vi "2023_day18.vi"() -> ()   [LabVIEW 2021]
panel:
  out "Task 2":i64
  out "Task 1 Data":cluster{i64[], i64[]}(graph)
  out "Task 2 Data":cluster{i64[], i64[]}(graph)
  out "Task 1":i64
  in  "Switch":bool caption="Ex. Data  vs.  User Data"
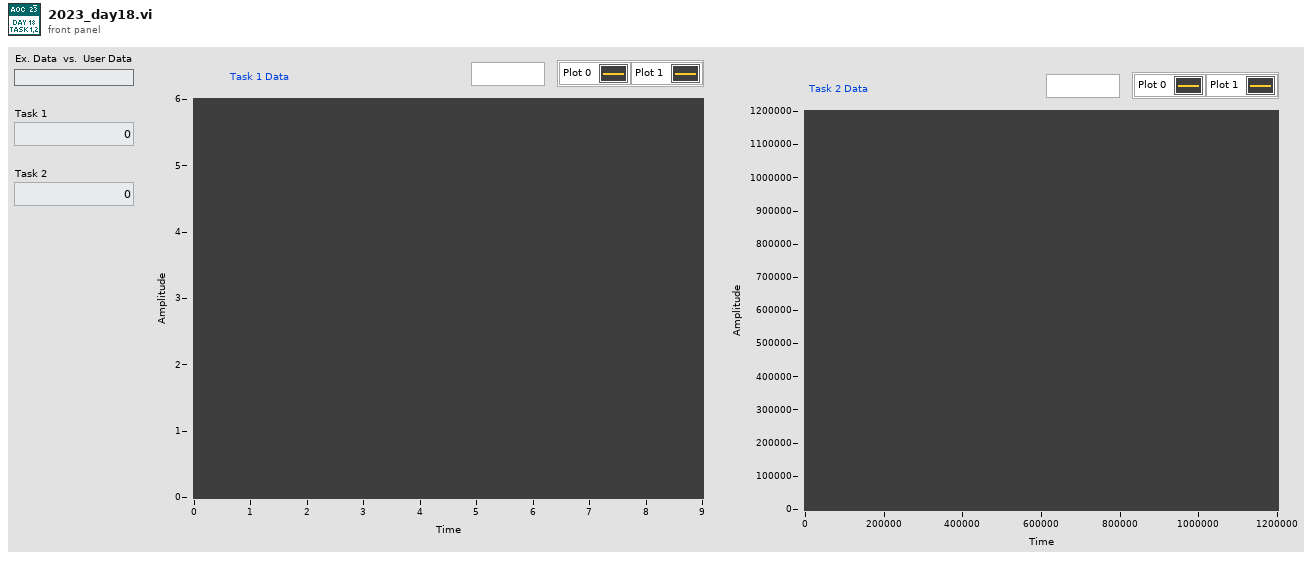
[diagram p1: front panel]
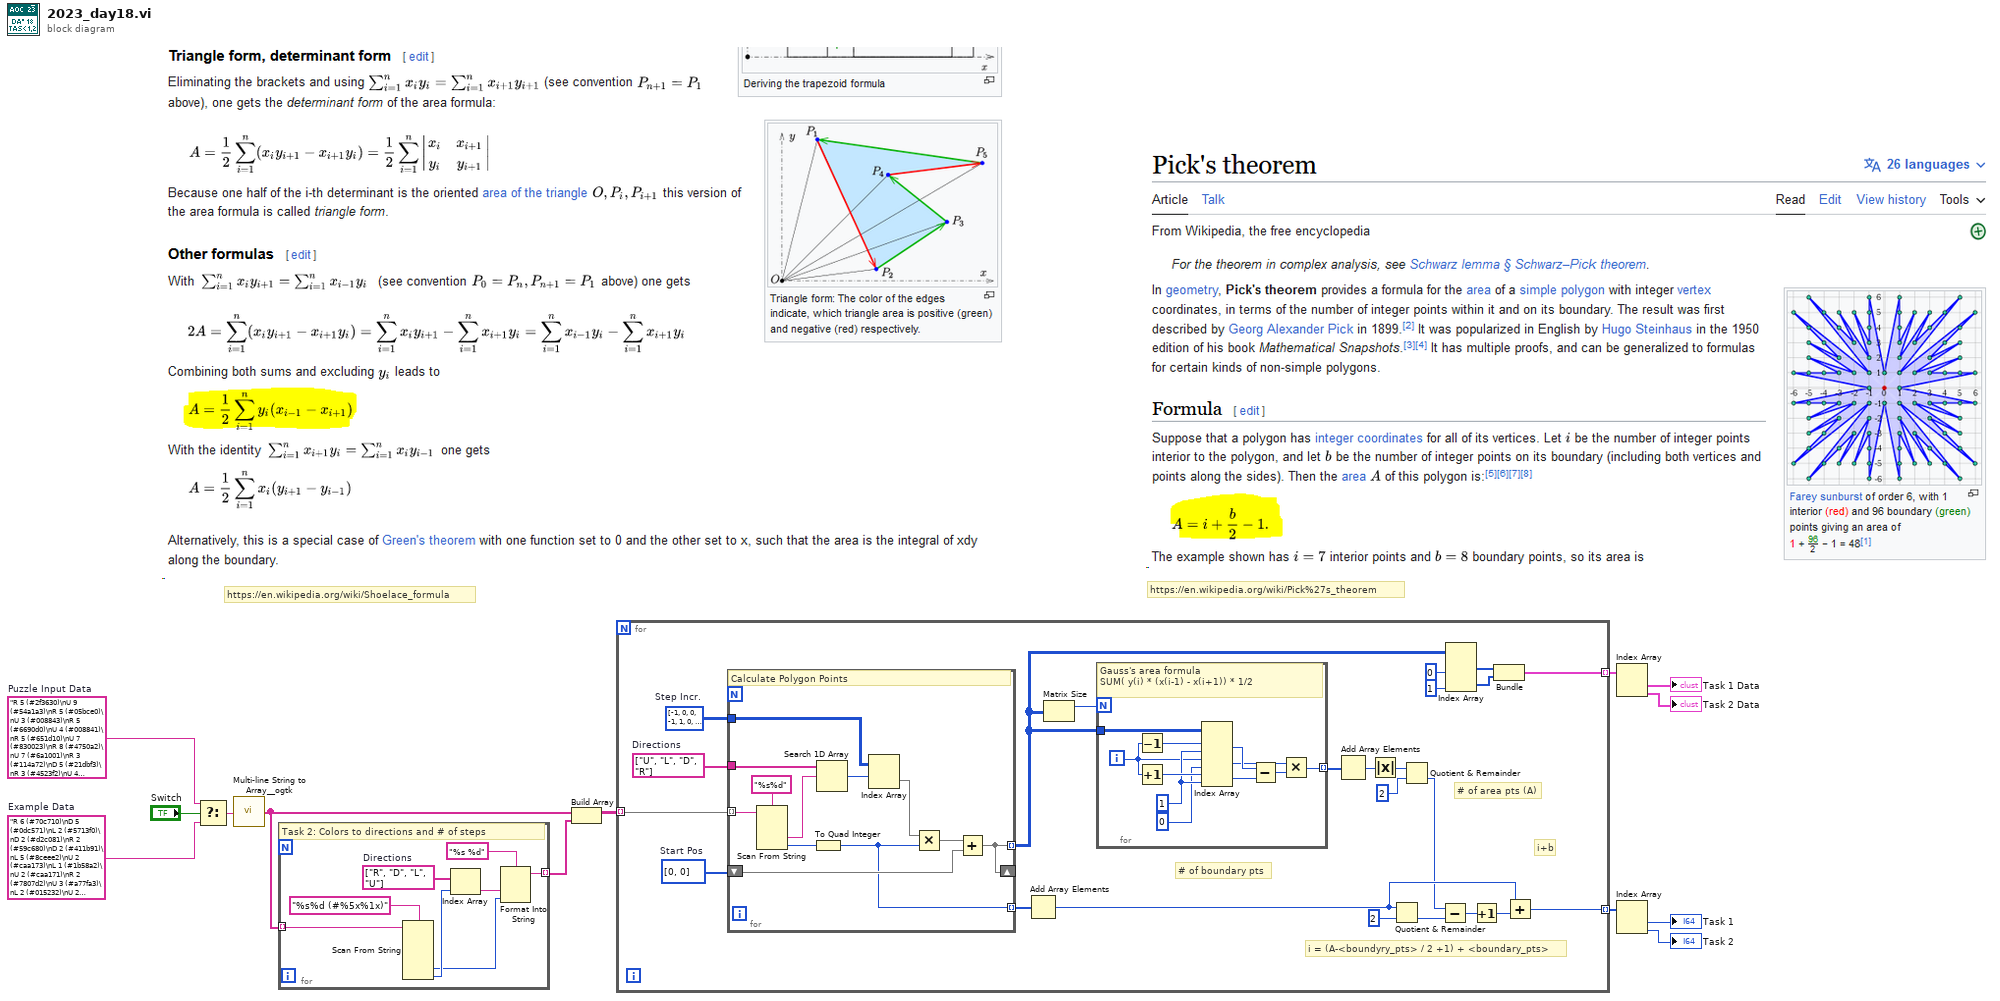
[diagram p0: block diagram]
diagram:
  w12 = "R 5 (#2f3630)\nU 9 (#54a1a3)\nR 5 (#05bce0)\nU 3 (#008843)\nR 5 (#6690d0)\nU 4 (#008841)\nR 5 (#651d10)\nU 7 (#830023)\nR 8 (#4750a2)\nU 7 (#6a1001)\nR 3 (#114a72)\nD 5 (#21dbf3)\nR 3 (#4523f2)\nU 4 (#3a1e43)\nR 4 (#2eef10)\nD 4 (#352183)\nR 5 (#2eef12)\nD 6 (#1fd943)\nL 7 (#5c0bd2)\nD 5 (#32d3b1)\nL 5 (#47d3d0)\nD 3 (#3032e1)\nR 2 (#47d3d2)\nD 4 (#4dee61)\nR 4 (#044a92)\nD 4 (#494b23)\nR 2 (#132772)\nD 3 (#2186a3)\nR 7 (#49e542)\nU 3 (#864783)\nR 3 (#3afdd2)\nU 5 (#2ab8d1)\nR 6 (#2d5072)\nD 5 (#362ab1)\nR 4 (#2d5070)\nU 5 (#46eaa1)\nR 9 (#183c12)\nU 3 (#494b21)\nR 3 (#584d32)\nU 4 (#6a1003)\nR 3 (#618682)\nU 4 (#5a1853)\nR 6 (#30cf00)\nU 6 (#6b3a23)\nR 5 (#5e1260)\nU 2 (#20b7d3)\nR 3 (#1d2ec0)\nU 10 (#89f613)\nR 5 (#16c5b0)\nU 3 (#26b1d3)\nR 4 (#475e70)\nU 3 (#007223)\nR 5 (#3cf870)\nU 3 (#851f83)\nR 8 (#326e40)\nU 5 (#043ad3)\nR 4 (#2eb0a0)\nU 5 (#26e791)\nR 3 (#0b6950)\nU 7 (#323af1)\nL 3 (#0b6952)\nU 3 (#4ffc41)\nL 4 (#721f70)\nU 8 (#0137b1)\nR 4 (#5c9d22)\nU 3 (#55ff21)\nR 5 (#5c9d20)\nU 3 (#3b2d71)\nR 5 (#721f72)\nU 7 (#1fa921)\nR 8 (#3012f0)\nD 5 (#4c6a91)\nR 8 (#61af70)\nD 4 (#4c6a93)\nR 6 (#2e21b0)\nD 2 (#7df243)\nR 2 (#108f72)\nD 9 (#239da3)\nR 5 (#1f8fb0)\nD 8 (#8e8b71)\nR 5 (#5a6f50)\nD 2 (#8e8b73)\nR 3 (#159190)\nD 5 (#5f70a3)\nL 5 (#012372)\nD 3 (#04bf23)\nL 5 (#72bbe2)\nD 6 (#04bf21)\nL 3 (#1bb142)\nD 3 (#0f6693)\nL 4 (#108f70)\nD 6 (#0ecae3)\nL 6 (#407170)\nD 8 (#10ff11)\nL 7 (#18f910)\nD 6 (#10ff13)\nR 2 (#483d30)\nD 6 (#30a891)\nR 4 (#1ed8b0)\nD 5 (#688901)\nR 4 (#130de0)\nD 6 (#4d20e1)\nR 5 (#4b1000)\nU 7 (#877bf1)\nR 2 (#395410)\nU 4 (#877bf3)\nR 4 (#167f10)\nD 2 (#486f11)\nR 7 (#54e8d0)\nD 2 (#504301)\nR 2 (#8035e2)\nD 7 (#433471)\nR 3 (#8035e0)\nD 3 (#26cad1)\nR 3 (#4b3dc0)\nD 5 (#802d11)\nR 2 (#05af00)\nD 4 (#3b3f31)\nR 5 (#0dfed0)\nD 8 (#3b4341)\nL 6 (#489830)\nD 3 (#3b4343)\nL 3 (#4e0bd0)\nD 7 (#0f7fd1)\nR 6 (#1c6dd0)\nD 2 (#318d21)\nR 3 (#0cb8f2)\nD 6 (#68acd1)\nR 2 (#432822)\nD 3 (#218ee1)\nR 11 (#661ec2)\nU 3 (#218ee3)\nR 5 (#0b10d2)\nU 4 (#2233f1)\nL 3 (#2a5330)\nU 3 (#0df7d1)\nL 9 (#5ff680)\nU 4 (#2b9701)\nR 12 (#8b68d0)\nU 3 (#2b9703)\nL 5 (#086f10)\nU 7 (#1f1431)\nR 4 (#6937b0)\nU 5 (#2cce51)\nR 3 (#26cb50)\nD 8 (#3ee1c1)\nR 6 (#3c8a40)\nD 5 (#7e7211)\nR 7 (#7190e0)\nD 3 (#036101)\nR 6 (#6110b0)\nD 3 (#89da01)\nL 12 (#1f2cc0)\nD 3 (#2b7181)\nL 4 (#3942b0)\nD 5 (#10f821)\nL 2 (#61ae90)\nD 6 (#04dee1)\nL 6 (#2fc950)\nD 2 (#04dee3)\nL 8 (#353d90)\nD 4 (#1e21b1)\nL 3 (#46fa00)\nD 4 (#3ea393)\nR 5 (#5c2e32)\nD 5 (#361be3)\nR 6 (#2ddc12)\nU 4 (#4b1a83)\nR 6 (#135722)\nU 6 (#521483)\nR 9 (#7382b2)\nD 6 (#239da3)\nR 3 (#3ed420)\nD 4 (#3a0c73)\nR 6 (#5a68d0)\nD 3 (#76f053)\nL 5 (#244ec0)\nD 4 (#062573)\nL 8 (#053c50)\nD 5 (#0bfac3)\nR 3 (#123e30)\nD 7 (#21c2c3)\nR 6 (#0b11b0)\nD 3 (#6781f3)\nR 9 (#720e70)\nD 3 (#7ddd13)\nL 11 (#33d6f0)\nD 2 (#1b2d83)\nL 7 (#5f0280)\nD 5 (#579183)\nR 4 (#5f0282)\nD 6 (#5c9303)\nR 3 (#3c6770)\nD 4 (#2b6333)\nR 5 (#4f28a0)\nU 5 (#55d573)\nR 6 (#2b03a0)\nU 5 (#244bd3)\nR 5 (#644122)\nU 7 (#08ab63)\nR 7 (#232bc2)\nU 5 (#71f5e3)\nR 4 (#060d22)\nU 3 (#168c63)\nR 4 (#44efa2)\nD 3 (#17c163)\nR 9 (#2ed822)\nD 6 (#17c161)\nR 10 (#4b9682)\nD 6 (#168c61)\nR 6 (#1ab282)\nD 3 (#490b43)\nL 6 (#639022)\nD 4 (#447151)\nL 5 (#0596c0)\nU 4 (#2fba61)\nL 5 (#0596c2)\nD 4 (#201131)\nL 3 (#1f9c52)\nD 3 (#0c4a23)\nR 9 (#266412)\nD 3 (#68bea3)\nR 7 (#266410)\nD 4 (#1f3423)\nR 3 (#51d9c2)\nD 6 (#1f6633)\nR 8 (#7382b0)\nU 8 (#01fca3)\nR 7 (#3271f0)\nU 4 (#7ee903)\nR 6 (#581210)\nD 7 (#7ee901)\nR 2 (#12dd60)\nU 7 (#15a1a3)\nR 6 (#7c30f0)\nU 2 (#591961)\nR 3 (#69efd0)\nU 4 (#591963)\nL 9 (#32e7e0)\nU 3 (#574071)\nL 3 (#50c6a0)\nU 3 (#0be261)\nL 5 (#6ae5c0)\nU 3 (#5c08b1)\nL 3 (#7158d0)\nU 2 (#36fe01)\nL 4 (#325c22)\nU 9 (#305be1)\nR 3 (#325c20)\nU 2 (#36c0a1)\nR 3 (#1687d0)\nU 7 (#6e3d91)\nR 4 (#69abb2)\nU 4 (#0a66d1)\nR 4 (#3091a2)\nU 6 (#548a01)\nR 3 (#47a5c2)\nU 3 (#2a9553)\nR 5 (#795b32)\nU 3 (#2a9551)\nR 8 (#181b72)\nU 7 (#43b071)\nR 4 (#443e90)\nU 2 (#3926e1)\nR 4 (#6c3760)\nU 4 (#694dd3)\nR 6 (#4b1d30)\nU 3 (#032dd1)\nR 6 (#101060)\nU 4 (#032dd3)\nL 6 (#49c630)\nU 7 (#694dd1)\nL 2 (#1df000)\nU 3 (#2ff181)\nL 8 (#3617e2)\nD 6 (#3a3c41)\nL 3 (#51c8c2)\nD 4 (#5c01b1)\nL 11 (#0ca2b0)\nU 2 (#4333b1)\nL 3 (#812b52)\nU 8 (#6f4601)\nL 3 (#379b22)\nU 2 (#07d291)\nL 7 (#49e292)\nU 7 (#709721)\nL 4 (#1db7a2)\nU 8 (#58c9d1)\nL 6 (#52d210)\nU 5 (#64a341)\nL 3 (#1054c0)\nU 7 (#64a343)\nL 4 (#61a0b0)\nU 10 (#187211)\nL 4 (#5b9920)\nU 4 (#05d301)\nL 3 (#0c8ef0)\nU 8 (#09f161)\nL 4 (#7fa590)\nU 4 (#516f31)\nL 3 (#408e12)\nD 6 (#3ccd51)\nL 2 (#4ba672)\nD 10 (#1fb771)\nL 3 (#3d8200)\nU 8 (#195531)\nL 3 (#6bcfe0)\nU 9 (#484041)\nL 5 (#3ae112)\nU 5 (#6d6931)\nR 4 (#3ae110)\nU 7 (#05dd71)\nL 4 (#4c5332)\nU 6 (#5df683)\nL 10 (#3aebd2)\nU 3 (#5f3f53)\nL 3 (#815352)\nU 6 (#5f3f51)\nL 4 (#28ac32)\nU 4 (#5df681)\nR 4 (#3cb5e2)\nU 2 (#7662f1)\nR 4 (#322d10)\nU 8 (#1a81a3)\nR 5 (#3e2ba0)\nD 4 (#1a81a1)\nR 3 (#362bc0)\nD 6 (#3e19c1)\nR 5 (#234960)\nU 5 (#2d2853)\nR 7 (#56bab0)\nU 4 (#2d2851)\nR 8 (#4d6be0)\nU 5 (#5ad541)\nR 8 (#1d6e52)\nU 6 (#077851)\nL 7 (#45b722)\nU 3 (#077853)\nL 7 (#52cf22)\nU 4 (#07d441)\nR 7 (#77bb62)\nU 4 (#1a8641)\nR 7 (#4c1bf2)\nU 3 (#2ca611)\nR 3 (#18b8e2)\nD 3 (#57ff81)\nR 4 (#60c622)\nD 7 (#42e791)\nR 4 (#1a7550)\nD 6 (#2645b1)\nR 5 (#1a7552)\nD 8 (#4ea9d1)\nR 6 (#797f00)\nD 2 (#02b451)\nR 4 (#375b52)\nD 7 (#28c491)\nR 7 (#5e30f2)\nD 9 (#3f4341)\nL 7 (#11cf50)\nD 5 (#82e171)\nR 3 (#655ee0)\nD 3 (#189ea1)\nR 3 (#772e32)\nD 10 (#177941)\nR 4 (#06baa2)\nD 11 (#561461)\nR 2 (#5c8dd2)\nD 7 (#561463)\nR 6 (#36fc22)\nD 5 (#0cea13)\nR 2 (#4cc760)\nD 4 (#4dfe53)\nR 6 (#323630)\nU 9 (#566003)\nR 7 (#7efd92)\nD 9 (#40f433)\nR 6 (#080d32)\nD 8 (#6cf311)\nR 5 (#35bf72)\nD 3 (#3b7973)\nR 8 (#06a632)\nD 4 (#252293)\nR 4 (#06a630)\nD 5 (#35ed03)\nR 7 (#4d1cd2)\nD 2 (#4cf4f3)\nR 3 (#1dd4e2)\nD 3 (#2b92f3)\nR 4 (#117530)\nD 4 (#5ac883)\nR 12 (#117532)\nU 4 (#48ca43)\nR 7 (#708b12)\nD 5 (#068663)\nR 5 (#4247e2)\nD 7 (#704161)\nR 4 (#4b2b22)\nD 8 (#13ea71)\nR 4 (#699472)\nD 5 (#4d6551)\nR 5 (#8503c0)\nD 2 (#281c91)\nR 2 (#8503c2)\nD 9 (#33a0c1)\nL 5 (#4e8ad2)\nD 3 (#825f21)\nL 5 (#26aab2)\nD 8 (#097c71)\nL 6 (#169832)\nD 4 (#457031)\nL 7 (#8cee10)\nU 5 (#251221)\nL 3 (#71dce0)\nU 3 (#331751)\nL 6 (#7cfe10)\nD 5 (#617961)\nL 9 (#7cfe12)\nU 5 (#04b4d1)\nL 8 (#379ae0)\nD 8 (#0c88f1)\nL 4 (#0ee942)\nD 8 (#297c01)\nR 5 (#5a78a2)\nD 6 (#3db043)\nR 5 (#7eadd2)\nD 4 (#3db041)\nR 5 (#4e5622)\nD 2 (#381fa1)\nR 6 (#2cfd90)\nD 4 (#36bd23)\nR 3 (#4d18c0)\nD 4 (#36bd21)\nR 3 (#1a3d70)\nD 2 (#6644a1)\nR 12 (#868912)\nD 4 (#5cb351)\nR 3 (#868910)\nD 4 (#3b3501)\nR 5 (#1cddb0)\nD 4 (#4cc9b1)\nL 9 (#040250)\nD 6 (#38c721)\nL 7 (#23e920)\nD 3 (#08dde3)\nL 8 (#2c48f0)\nD 4 (#08dde1)\nL 2 (#414710)\nD 4 (#3c36b1)\nL 8 (#467ab0)\nD 3 (#034323)\nL 4 (#67f960)\nD 6 (#034321)\nL 9 (#675f90)\nD 6 (#338083)\nL 5 (#2b4702)\nD 6 (#035ab3)\nL 6 (#4d5642)\nD 7 (#035ab1)\nL 8 (#40ff22)\nD 3 (#495523)\nL 5 (#83a372)\nD 5 (#1a5d23)\nL 8 (#4ef3c2)\nD 4 (#7515a3)\nL 9 (#40d0f0)\nD 5 (#143e73)\nL 8 (#2ec480)\nU 8 (#070d81)\nR 4 (#344d10)\nU 4 (#070d83)\nR 5 (#2eb4b0)\nU 5 (#681243)\nR 3 (#51a710)\nU 5 (#8a2821)\nR 7 (#2faba0)\nU 5 (#8a2823)\nR 3 (#3849b0)\nU 6 (#375b63)\nL 8 (#3790d0)\nU 7 (#2f77d1)\nL 6 (#444dd0)\nU 3 (#85afe3)\nL 6 (#656d90)\nU 6 (#85afe1)\nL 2 (#1152b0)\nU 3 (#334491)\nR 4 (#362670)\nU 7 (#819361)\nL 4 (#4fd202)\nU 3 (#718a21)\nL 5 (#17bf92)\nD 10 (#3334f1)\nL 2 (#43c272)\nD 4 (#40f041)\nL 5 (#3afbc2)\nD 6 (#742533)\nL 8 (#0ae4c2)\nU 6 (#146731)\nL 8 (#2aec82)\nD 2 (#89fa61)\nL 3 (#044562)\nD 4 (#1e14a1)\nR 2 (#7b0a82)\nD 4 (#1e14a3)\nR 7 (#4b7812)\nD 2 (#09cdc1)\nR 5 (#3c3502)\nD 2 (#70eb41)\nR 12 (#4b7400)\nD 3 (#5c8043)\nL 12 (#6085c0)\nD 3 (#5c8041)\nL 4 (#5b0330)\nD 4 (#74bce1)\nL 12 (#6f6142)\nD 2 (#0f2211)\nL 5 (#40e5b0)\nD 5 (#72afc1)\nL 7 (#40e5b2)\nD 3 (#160a51)\nL 3 (#7a6c72)\nD 6 (#3ade81)\nL 4 (#6c12d2)\nU 10 (#0d3851)\nL 5 (#4e1680)\nD 10 (#65ba61)\nL 5 (#185f10)\nD 3 (#65ba63)\nL 6 (#3ca040)\nD 7 (#6970e1)\nL 3 (#49ad52)\nD 2 (#0c8481)\nL 8 (#3e7a82)\nD 3 (#0c8483)\nL 5 (#1aee02)\nD 4 (#35e721)\nL 4 (#39f672)\nD 5 (#07f333)\nL 6 (#730842)\nD 6 (#0fe7b3)\nL 3 (#6079e2)\nD 9 (#74e4d3)\nL 7 (#6079e0)\nD 4 (#1c77b3)\nL 3 (#3299b2)\nU 4 (#6649e3)\nL 5 (#496642)\nU 5 (#618563)\nL 4 (#36e332)\nD 4 (#084843)\nL 6 (#670e22)\nD 9 (#164f23)\nL 5 (#3c5360)\nD 5 (#467003)\nL 3 (#3c5362)\nU 3 (#3980d3)\nL 3 (#275e32)\nU 6 (#19ea63)\nL 4 (#855df0)\nU 2 (#5ec993)\nL 9 (#66f342)\nU 7 (#4ac7a3)\nL 5 (#1e6ab2)\nU 8 (#2bd3a3)\nL 4 (#5f6272)\nU 5 (#3b2031)\nL 4 (#1c1fa0)\nU 5 (#534711)\nR 3 (#1c1fa2)\nU 5 (#3474d1)\nR 5 (#572be2)\nD 4 (#2cdf53)\nR 6 (#3bb0e2)\nU 4 (#5e9073)\nR 4 (#3bb0e0)\nU 4 (#376c53)\nL 3 (#193f72)\nU 3 (#484e83)\nL 4 (#799b82)\nU 5 (#52f273)\nR 4 (#376190)\nU 5 (#3650a3)\nL 5 (#7def10)\nD 2 (#20fa83)\nL 2 (#089240)\nD 11 (#49c3a3)\nL 3 (#768be0)\nU 4 (#42fa23)\nL 5 (#5ab362)\nU 4 (#593983)\nL 8 (#5e6ba2)\nD 4 (#593981)\nR 4 (#7b4fc2)\nD 9 (#44a9c3)\nL 2 (#086692)\nD 3 (#7ce9f3)\nL 4 (#68b430)\nU 6 (#5ab7c1)\nL 4 (#430330)\nD 6 (#0b1593)\nL 5 (#1ca4a0)\nD 5 (#0b1591)\nR 10 (#429f80)\nD 2 (#5ab7c3)\nR 2 (#292be0)\nD 4 (#7a8693)\nR 3 (#12dfd2)\nD 10 (#2244f3)\nL 4 (#4eeb62)\nD 10 (#4831c3)\nL 6 (#25aa50)\nU 8 (#379b33)\nL 3 (#25aa52)\nU 3 (#145863)\nL 5 (#480492)\nU 4 (#69feb1)\nL 7 (#593592)\nU 4 (#4c6b91)\nL 5 (#312212)\nU 3 (#26df43)\nR 12 (#68b362)\nU 4 (#6e94f3)\nL 5 (#28bd52)\nU 4 (#1aea03)\nL 8 (#615f22)\nU 2 (#6fb163)\nL 2 (#40b8a2)\nU 7 (#09d633)\nL 7 (#044e02)\nU 8 (#1a4333)\nL 4 (#172d00)\nU 2 (#4509c3)\nL 6 (#4de1d0)\nU 7 (#818a41)\nL 4 (#0ce4b0)\nU 7 (#0745d1)\nR 6 (#520370)\nU 2 (#5a7db3)\nR 8 (#2f93c0)\nU 4 (#2e5263)\nL 4 (#147e00)\nU 3 (#44d303)\nL 7 (#245640)\nU 4 (#17d933)\nL 3 (#4f6820)\nU 3 (#17d931)\nL 10 (#488c50)\nD 3 (#108b33)\nL 4 (#300e60)\nD 3 (#887d43)\nR 7 (#4272d0)\nD 8 (#657091)\nL 7 (#63d120)\nD 3 (#230cb1)\nR 4 (#04e1b0)\nD 6 (#4ba9a3)\nL 7 (#055c40)\nU 2 (#3ee173)\nL 4 (#454062)\nU 6 (#2af563)\nL 3 (#40a642)\nU 6 (#4ddf13)\nL 6 (#85e6a0)\nU 6 (#090df3)\nL 9 (#055c42)\nU 2 (#4ac2b3)\nL 3 (#2ae1a0)\nU 5 (#43af51)\nR 6 (#860900)\nU 5 (#43af53)\nL 6 (#057bb0)\nU 3 (#570c13)\nR 4 (#515d92)\nU 3 (#09a031)\nL 7 (#45b7f2)\nU 5 (#09a033)\nR 6 (#1f50d2)\nU 7 (#4e6373)\nL 6 (#5df030)\nU 7 (#004663)\nR 7 (#10f120)\nU 4 (#5f4883)\nL 12 (#10f122)\nU 2 (#441aa3)\nL 3 (#1c7242)\nU 4 (#4849a3)\nR 7 (#7026d2)\nU 4 (#442943)\nR 8 (#5c5152)\nU 5 (#563813)\nL 4 (#5c5150)\nU 4 (#1460b3)\nL 5 (#1d3272)\nU 6 (#1d15d3)\nR 5 (#4fe282)\nU 3 (#6a04c1)\nL 6 (#2ca912)\nU 5 (#1d2623)\nL 6 (#298bb2)\nU 3 (#1d2621)\nL 9 (#3a4e82)\nU 4 (#2abf71)\nL 5 (#01c5d2)\nU 4 (#7f5d41)\nL 6 (#0149b2)\nU 4 (#66f8c3)\nL 5 (#53acd2)\nU 6 (#55caa3)\nL 3 (#676e82)\nU 8 (#5c69a3)\nR 5 (#5d7ed2)\nU 2 (#1d90a3)\nR 3 (#579cb2)\nU 3 (#631003)\nR 9 (#6ffcb2)\nU 5 (#2e98f3)\nR 2 (#036c22)\nU 3 (#2bd763)\nL 5 (#478442)\nU 7 (#7a8373)\nL 9 (#5da862)\nU 4 (#13a8d3)"  # Puzzle Input Data
  w10 = "R 6 (#70c710)\nD 5 (#0dc571)\nL 2 (#5713f0)\nD 2 (#d2c081)\nR 2 (#59c680)\nD 2 (#411b91)\nL 5 (#8ceee2)\nU 2 (#caa173)\nL 1 (#1b58a2)\nU 2 (#caa171)\nR 2 (#7807d2)\nU 3 (#a77fa3)\nL 2 (#015232)\nU 2 (#7a21e3)"  # Example Data
  # "https://en.wikipedia.org/wiki/Shoelace_formula"
  # "https://en.wikipedia.org/wiki/Pick%27s_theorem"
  n1 = Select(t=w12, s="Switch", f=w10) -> (s? t:f=w11:string)
  n2 = call <userlib>:"Multi-line String to Array__ogtk.vi"("string"=w11) -> ("lines"=w9:string[])
  n3 = for {
    tunnel: [w14] -> w7 mode=indexing
    tunnel: w9 -> [w21] mode=indexing
    w18 = string[] ["R", "D", "L", "U"]  # Directions
    # "Task 2: Colors to directions and # of steps"
    n4 = Scan From String(format string="%s%d (#%5x%1x)", input string=w21) -> (output 3=w15:u32, output 4=w19:u32)  [unwired: 8 in, 3 out]
    n5 = Index Array(array=w18, index=w19) -> (element=w16:string)
    n6 = Format Into String(format string="%s %d", w16, w15) -> (resulting string=w14:string)  [unwired: 2 in, 1 out]
  }
  n7 = Build Array(w9, w7) -> (w8:string[][])
  n8 = for {
    tunnel: w8 -> [w35] mode=indexing
    tunnel: [w23] -> w6 mode=indexing
    tunnel: [w22] -> w3 mode=indexing
    w33 = i64[] [0, 0]  # Start Pos
    w43 = i64[][] [[-1, 0], [0, -1], [1, 0], [0, 1]]  # Step Incr.
    w44 = string[] ["U", "L", "D", "R"]  # Directions
    # "i+b"
    # "i = (A-<boundyry_pts> / 2 +1) + <boundary_pts>"
    # "# of boundary pts"
    # "# of area pts (A)"
    n9 = for {
      tunnel: w44 -> [w52]
      tunnel: w43 -> [w51]
      shift-right: [w45] -> _
      shift-left: w33 -> [w54]
      tunnel: [w46] -> w34 mode=indexing
      tunnel: w35 -> [w47] mode=indexing
      tunnel: [w45] -> w25 mode=indexing
      # "Calculate Polygon Points"
      n10 = Scan From String(format string="%s%d", input string=w47) -> (output 1=w53:string, output 2=w48:i32)  [unwired: 4 in, 3 out]
      n11 = To Quad Integer(1:w48) -> (0:w46:i64)
      n12 = Search 1D Array(1D array=w52, element=w53) -> (index of element=w55:i32)  [unwired: 1 in]
      n13 = Index Array(array=w51, index (row)=w55) -> (element=w50:i64[])  [unwired: 1 in]
      n14 = Multiply(x=w50, y=w46) -> (x*y=w49:i64[])
      n15 = Add(x=w49, y=w54) -> (x+y=w45:i64[])
    }
    n16 = Add Array Elements(numeric array=w34) -> (sum=w26:i64)
    n17 = Matrix Size(0:w25) -> (1:w42:i32)  [unwired: 1 out]
    n18 = for {
      N: w42 -> [_]
      tunnel: w25 -> [w67]
      tunnel: [w57] -> w28 mode=indexing
      i -> [w59]
      w64 = 1 ("disabled index (col)")
      # "Gauss's area formula\nSUM( y(i) * (x(i-1) - x(i+1)) * 1/2"
      n19 = Decrement(x=w59) -> (x-1=w66:i32)
      n20 = Increment(x=w59) -> (x+1=w65:i32)
      n21 = Index Array(array=w67, index (row) #1=w66, index (col) #1=w64, index (row) #2=w59, index (col) #2=0 ("disabled index (col)"), index (row) #3=w65, index (col) #3=w64) -> (element #1=w62:i64, element #2=w58:i64, element #3=w60:i64)
      n22 = Subtract(x=w62, y=w60) -> (x-y=w61:i64)
      n23 = Multiply(x=w58, y=w61) -> (x*y=w57:i64)
    }
    n24 = Add Array Elements(numeric array=w28) -> (sum=w27:i64)
    n25 = Absolute Value(x=w27) -> (abs(x)=w36:i64)
    n26 = Quotient & Remainder(x=w26, y=i64 2) -> (floor(x/y)=w39:i64)  [unwired: 1 out]
    n27 = Quotient & Remainder(x=w36, y=i64 2) -> (floor(x/y)=w24:i64)  [unwired: 1 out]
    n28 = Subtract(x=w24, y=w39) -> (x-y=w38:i64)
    n29 = Index Array(array=w25, index (col) #1=0 ("disabled index (col)"), index (col) #2=1 ("disabled index (col)")) -> (element #1=w30:i64[], element #2=w29:i64[])  [unwired: 2 in]
    n30 = Increment(x=w38) -> (x+1=w37:i64)
    n31 = Bundle(w30, w29) -> (w23:cluster{i64[], i64[]})  [unwired: 1 in]
    n32 = Add(x=w26, y=w37) -> (x+y=w22:i64)
  }
  n33 = Index Array(array=w6) -> (element #1=→"Task 1 Data":cluster{i64[], i64[]}, element #2=→"Task 2 Data":cluster{i64[], i64[]})  [unwired: 2 in]
  n34 = Index Array(array=w3) -> (element #1=→"Task 1":i64, element #2=→"Task 2":i64)  [unwired: 2 in]
